vi "JSONtext Tree VI.vi"   [LabVIEW 2017]
uses:
  JSONtext.lvlib
  Find Object Item (single) by Path.vi
  From JSON Text (string).vi
  Insert into Object.vi
  b8bde55b-cc7e-4f15-aea1-72f916afde05.vi
  JSON Value Type.ctl
types:
  T1 = typedef "JSONtext.lvlib/JSON Value Type.ctl" = enum16{"Not a JSON Value", "JSON Object", "JSON Array", "String", "Number", "true", "false", "null"}
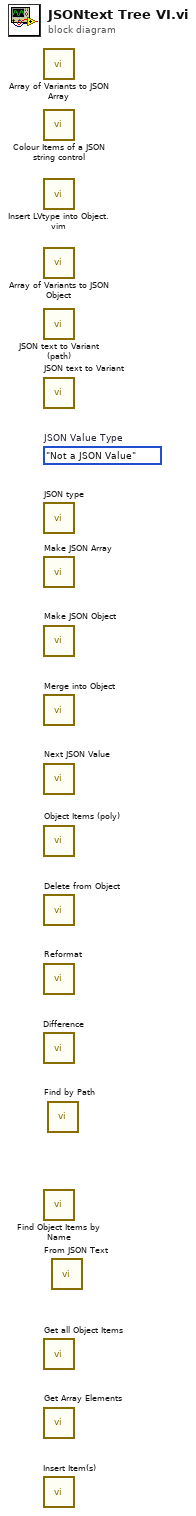
[diagram p0: block diagram]
diagram:
  (unwired) JSON_Value_Type."Not a JSON Value"  # JSON Value Type
  n1 = call "Array of Variants to JSON Array.vi"() -> ()  [unwired: 10 in, 2 out]
  n2 = call "Colour Items of a JSON string control.vi"() -> ()  [unwired: 12 in]
  n3 = call "Insert LVtype into Object.vim"() -> ()  [unwired: 8 in, 3 out]
  n4 = call "Array of Variants to JSON Object.vi"() -> ()  [unwired: 10 in, 2 out]
  n5 = call "JSON text to Variant (path).vi"() -> ()  [unwired: 9 in, 3 out]
  n6 = call "JSON text to Variant.vi"() -> ()  [unwired: 10 in, 2 out]
  n7 = call "JSON type.vi"() -> ()  [unwired: 10 in, 2 out]
  n8 = call "Make JSON Array.vi"() -> ()  [unwired: 10 in, 2 out]
  n9 = call "Make JSON Object.vi"() -> ()  [unwired: 10 in, 2 out]
  n10 = call "Merge into Object.vi"() -> ()  [unwired: 9 in, 2 out]
  n11 = call "Next JSON Value.vi"() -> ()  [unwired: 8 in, 4 out]
  n12 = call-poly "Object Items (poly).vi"() -> ()  [unwired: 9 in, 3 out]
  n13 = call "Delete from Object.vi"() -> ()  [unwired: 7 in, 4 out]
  n14 = call "Reformat.vi"() -> ()  [unwired: 8 in, 4 out]
  n15 = call "Difference.vi"() -> ()  [unwired: 9 in, 2 out]
  n16 = call "Find Object Items by Name.vi"() -> ()  [unwired: 9 in, 3 out]
  n17 = call "Get all Object Items.vi"() -> ()  [unwired: 8 in, 4 out]
  n18 = call "Get Array Elements.vi"() -> ()  [unwired: 9 in, 3 out]
  n19 = call-poly "Insert Item(s).vi"() -> ()  [unwired: 8 in, 3 out]
  n20 = call-poly "Find by Path.vi"() -> ()  [unwired: 8 in, 4 out]
  n21 = call-poly "From JSON Text.vi"() -> ()  [unwired: 9 in, 3 out]
